vi "Add NI-XNET CAN Hardware_Add Log File.vi"(7 "SysDef Ref":T1, 8 "error in (no error)":errorcluster, 9 "Log Files":T2[](array[typedef]) {"Operation" items=["ContinueLoggingInNewFile", "StopLogging"]; "LimitType" items=["Footprint", "Time"]; "TriggerType" items=["StartLoggingOnNonZero", "StartLoggingOnZero", "EnableLoggingWhenTriggerIsZero", "EnableLoggingWhenTriggerIsNonZero"]; "Filter" items=["LogEntireBusTraffic", "ExcludeFrameIDs", "IncludeFrameIDs"]; "DataLoggingFileType" items=["TDMS", "NCL"]}, 11 "CAN Port Ref":refnum<k24>) -> (0 "error out":errorcluster, 3 "CAN Port Ref out":refnum<k24>)   [LabVIEW 2019, in "Simple SysDef API.lvlib"]
uses:
  <userlib>/SimpleSysDef/Simple SysDef API.lvlib
  <userlib>/SimpleSysDef/_SubVIs/Add NI-XNET CAN Hardware_Add Log File_Settings.ctl
  <userlib>/SimpleSysDef/_SubVIs/System Definition Reference.ctl
  NationalInstruments.VeriStand.SystemDefinitionAPI
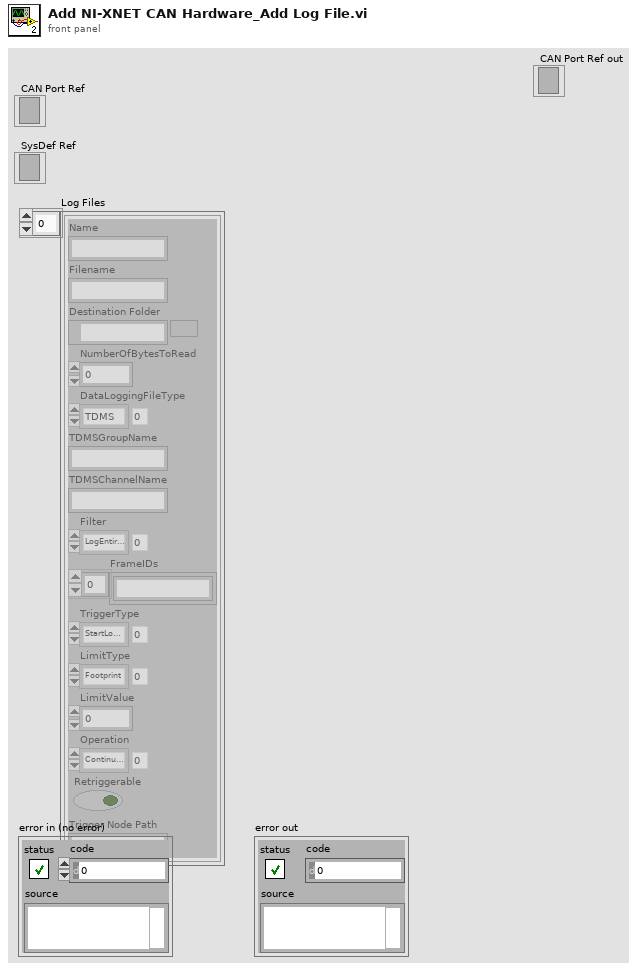
[diagram p1: front panel]
types:
  T1 = typedef "Simple SysDef API.lvlib/System Definition Reference.ctl" = refnum<k24>
  T2 = typedef "Simple SysDef API.lvlib/Add NI-XNET CAN Hardware_Add Log File_Settings.ctl" = cluster{"Name":string, "Filename":string, "Destination Folder":path, "NumberOfBytesToRead":u32, "DataLoggingFileType":i32, "TDMSGroupName":string, "TDMSChannelName":string, "Filter":i32, "FrameIDs":string[], "TriggerType":i32, "LimitType":i32, "LimitValue":u32, "Operation":i32, "Retriggerable":bool, "Trigger Node Path":string}
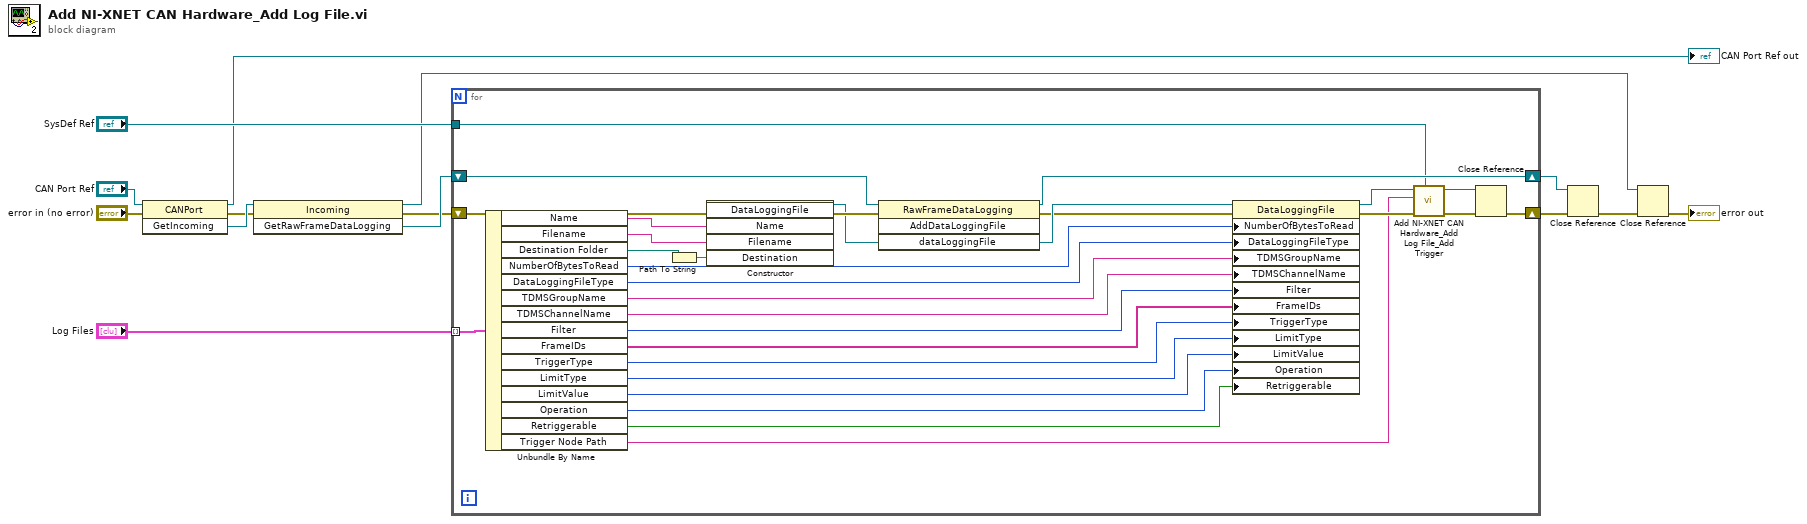
[diagram p0: block diagram]
diagram:
  n1 = invoke class="CANPort" method="GetIncoming"(reference="CAN Port Ref", error in="error in (no error)") -> (reference out=→"CAN Port Ref out":refnum<k24>, error out=w7:errorcluster, "GetIncoming"=w10:refnum<k24>)  [unwired: 1 in]
  n2 = invoke class="Incoming" method="GetRawFrameDataLogging"(reference=w10, error in=w7) -> (reference out=w6:refnum<k24>, error out=w8:errorcluster, "GetRawFrameDataLogging"=w9:refnum<k24>)  [unwired: 1 in]
  n3 = for {
    shift-right: [w40] -> w3
    shift-left: w8 -> [w42]
    shift-right: [w41] -> w5
    shift-left: w9 -> [w39]
    tunnel: "SysDef Ref" -> [w34]
    tunnel: "Log Files" -> [w33] mode=indexing
    n4 = Unbundle By Name(w33) -> ("Name"=w32:string, "Filename"=w31:string, "Destination Folder"=w30:path, "NumberOfBytesToRead"=w26:u32, "DataLoggingFileType"=w25:i32, "TDMSGroupName"=w24:string, "TDMSChannelName"=w23:string, "Filter"=w22:i32, "FrameIDs"=w21:string[], "TriggerType"=w20:i32, "LimitType"=w19:i32, "LimitValue"=w18:u32, "Operation"=w17:i32, "Retriggerable"=w16:bool, "Trigger Node Path"=w15:string)
    n5 = Path To String(path=w30) -> (string=w29:string)
    n6 = constructor class="DataLoggingFile"(error in=w42, "Name"=w32, "Filename"=w31, "Destination"=w29) -> (reference out=w38:refnum<k24>, error out=w43:errorcluster)  [unwired: 2 in, 4 out]
    n7 = invoke class="RawFrameDataLogging" method="AddDataLoggingFile"(reference=w39, error in=w43, "dataLoggingFile"=w38) -> (reference out=w41:refnum<k24>, error out=w28:errorcluster)  [unwired: 1 in, 2 out]
    n8 = property class="DataLoggingFile"(reference=w38, error in=w28, "NumberOfBytesToRead"=w26, "DataLoggingFileType"=w25, "TDMSGroupName"=w24, "TDMSChannelName"=w23, "Filter"=w22, "FrameIDs"=w21, "TriggerType"=w20, "LimitType"=w19, "LimitValue"=w18, "Operation"=w17, "Retriggerable"=w16) -> (reference out=w37:refnum<k24>, error out=w27:errorcluster)
    n9 = call <userlib>:"Add NI-XNET CAN Hardware_Add Log File_Add Trigger.vi"("SysDef Ref"=w34, "error in (no error)"=w27, "Trigger Node Path"=w15, "Log File Ref"=w37) -> ("error out"=w35:errorcluster, "Log File Ref out"=w36:refnum<k24>)  [unwired: 6 in]
    n10 = Close Reference(reference=w36, error in (no error)=w35) -> (error out=w40:errorcluster)
  }
  n11 = Close Reference(reference=w5, error in (no error)=w3) -> (error out=w4:errorcluster)
  n12 = Close Reference(reference=w6, error in (no error)=w4) -> (error out=→"error out":errorcluster)
